vi "Splash.vi"() -> ()   [LabVIEW 2013]
panel:
  out "Contour Plot":picture
  # "Initializing Demo..."
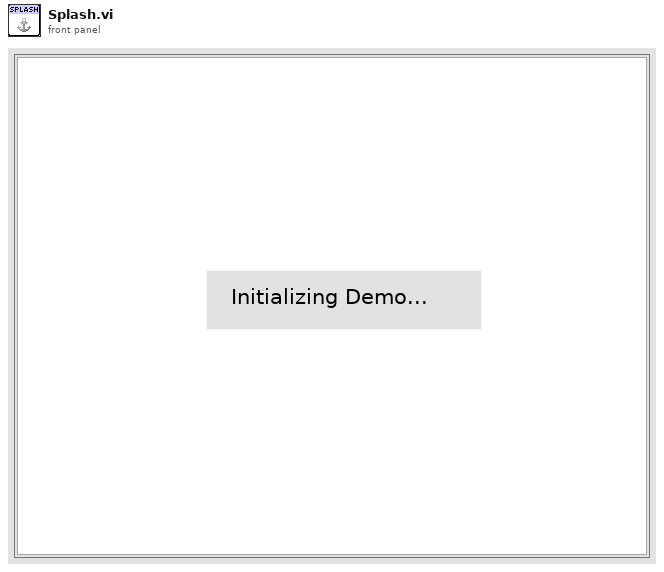
[diagram p1: front panel]
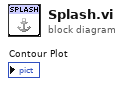
[diagram p0: block diagram]
diagram:
